vi "test_libssh2_sftp_statvfs.vi"() -> ()   [LabVIEW 2017, in "integration_tests.lvlib"]
uses:
  integration_tests.lvlib
  support/support.lvlib
  libssh2/libssh2.lvlib
  <vilib>/PNR/Transparent Assertions/Transparent Assertions/Transparent Assertions.lvlib
panel:
  out "error out":errorcluster
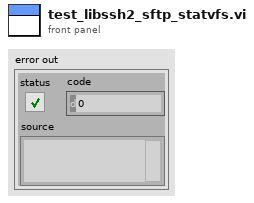
[diagram p1: front panel]
types:
  T1 = typedef "libssh2.lvlib/Session Refnum.ctl" = refnum<k1>
  T2 = typedef "libssh2.lvlib/SFTP Refnum.ctl" = refnum<k1>
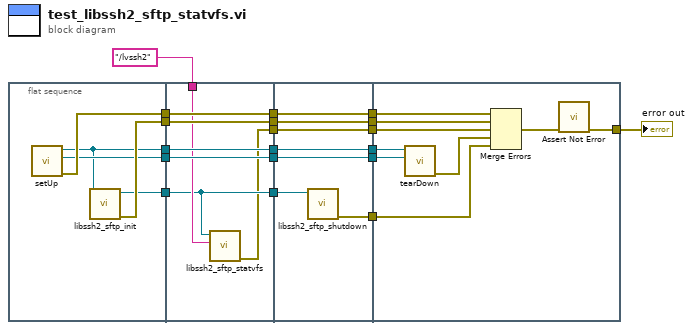
[diagram p0: block diagram]
diagram:
  n1 = flat-sequence {
    tunnel: [w24] -> w12
    tunnel: [w23] -> w11
    tunnel: [w22] -> w10
    tunnel: [w21] -> w9
    tunnel: [w20] -> w8
    tunnel: w12 -> [w31]
    tunnel: [w31] -> w7
    tunnel: w11 -> [w30]
    tunnel: [w30] -> w6
    tunnel: w10 -> [w26]
    tunnel: [w26] -> w5
    tunnel: w9 -> [w29]
    tunnel: [w29] -> w4
    tunnel: w8 -> [w28]
    tunnel: [w28] -> w3
    tunnel: "/lvssh2" ("filename") -> [w27]
    tunnel: [w25] -> w2
    tunnel: w3 -> [w38]
    tunnel: [w38] -> w18
    tunnel: w4 -> [w37]
    tunnel: [w37] -> w17
    tunnel: w5 -> [w34]
    tunnel: w6 -> [w36]
    tunnel: [w36] -> w16
    tunnel: w7 -> [w35]
    tunnel: [w35] -> w15
    tunnel: [w33] -> w14
    tunnel: w2 -> [w32]
    tunnel: [w32] -> w1
    tunnel: w18 -> [w47]
    tunnel: w17 -> [w46]
    tunnel: w16 -> [w45]
    tunnel: [w40] -> w19
    tunnel: w15 -> [w42]
    tunnel: w14 -> [w41]
    tunnel: w1 -> [w39]
    frame #0 {
      n2 = call "setUp.vi"() -> ("error out"=w23:errorcluster, "connection ID"=w21:refnum<k5>, "session"=w20:T1)  [unwired: 9 in]
      n3 = call "libssh2_sftp_init.vi"("session"=w20) -> ("error out"=w24:errorcluster, "sftp"=w22:T2)  [unwired: 9 in]
    }
    frame #1 {
      n4 = call "libssh2_sftp_statvfs.vi"("path"=w27, "sftp"=w26) -> ("error out"=w25:errorcluster)  [unwired: 8 in, 1 out]
    }
    frame #2 {
      n5 = call "libssh2_sftp_shutdown.vi"("sftp"=w34) -> ("error out"=w33:errorcluster)  [unwired: 10 in]
    }
    frame #3 {
      n6 = call "tearDown.vi"("connection ID"=w46, "session"=w47) -> ("error out"=w44:errorcluster)  [unwired: 9 in]
      n7 = Merge Errors(w45, w42, w39, w44, w41) -> (w43:errorcluster)
      n8 = call <vilib>:"Assert Not Error.vi"("error in (no error)"=w43) -> ("error out"=w40:errorcluster)  [unwired: 10 in]
    }
  }
  "error out" <- w19
